vi "Global.vi"() -> ()   [LabVIEW 2019]
panel:
  out "TIRF-LockIsCalbrated?":bool
  out "TirfLockPrintArray":cluster{"X":dbl, "Y":dbl}[](array[cluster])
  in  "TirfLockPrintCounter":dbl
  out "LasersForAlignment":bool
  in  "MouseDownY":dbl
  in  "MouseDownX":dbl
  out "MouseDownWithinImage":bool
  in  "Debug":bool
  # "On"
  # "Off"
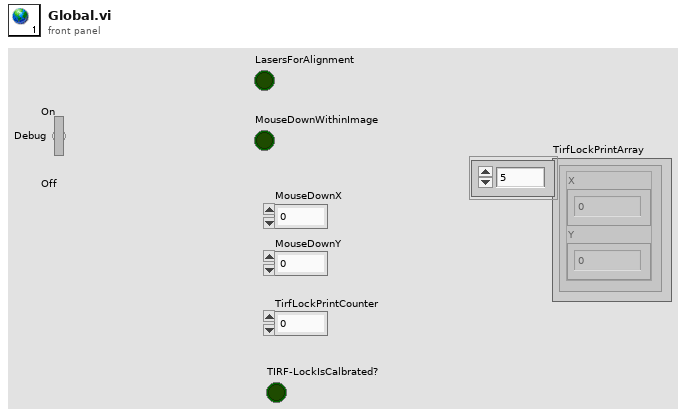
[diagram p1: front panel]
diagram:
